vi "串口上位机.vi"() -> ()   [LabVIEW 2011]
uses:
  <vilib>/Utility/error.llb/whitespace.ctl
  <vilib>/Instr/_visa.llb/VISA Configure Serial Port (Instr).vi
  <vilib>/Utility/file.llb/Write To Spreadsheet File (string).vi
panel:
  out "提示灯":bool
  out "连接的字符串":string
  out "心率记录表":string[][](table)
  in  "心率文档存放路径":path
  out "错误输出":errorcluster
  out "接收手机端内容显示区":string
  out "错误输出 2":errorcluster caption="错误输出"
  in  "停止":bool
  out "心率显示":i32
  in  "确定按钮":dbl
  out "error out":errorcluster caption="错误输出"
  out "滑动杆":T1 scale=0.0..10.0
  out "发送记录":string
  out "发送总字节数":u32
  out "发送字节数":u32
  out "发送错误状态":bool
  in  "发送":bool
  out "接收内容":string
  in  "发送内容":string
  out "工作状态":bool
  in  "baud rate (9600)":u32=115200 caption="波特率"
  in  "串口号":refnum<visa-resource-name>
  in  "关闭串口":bool
  in  "打开串口":bool
  # "嵌入式设备通信区"
  # "物联网通信区"
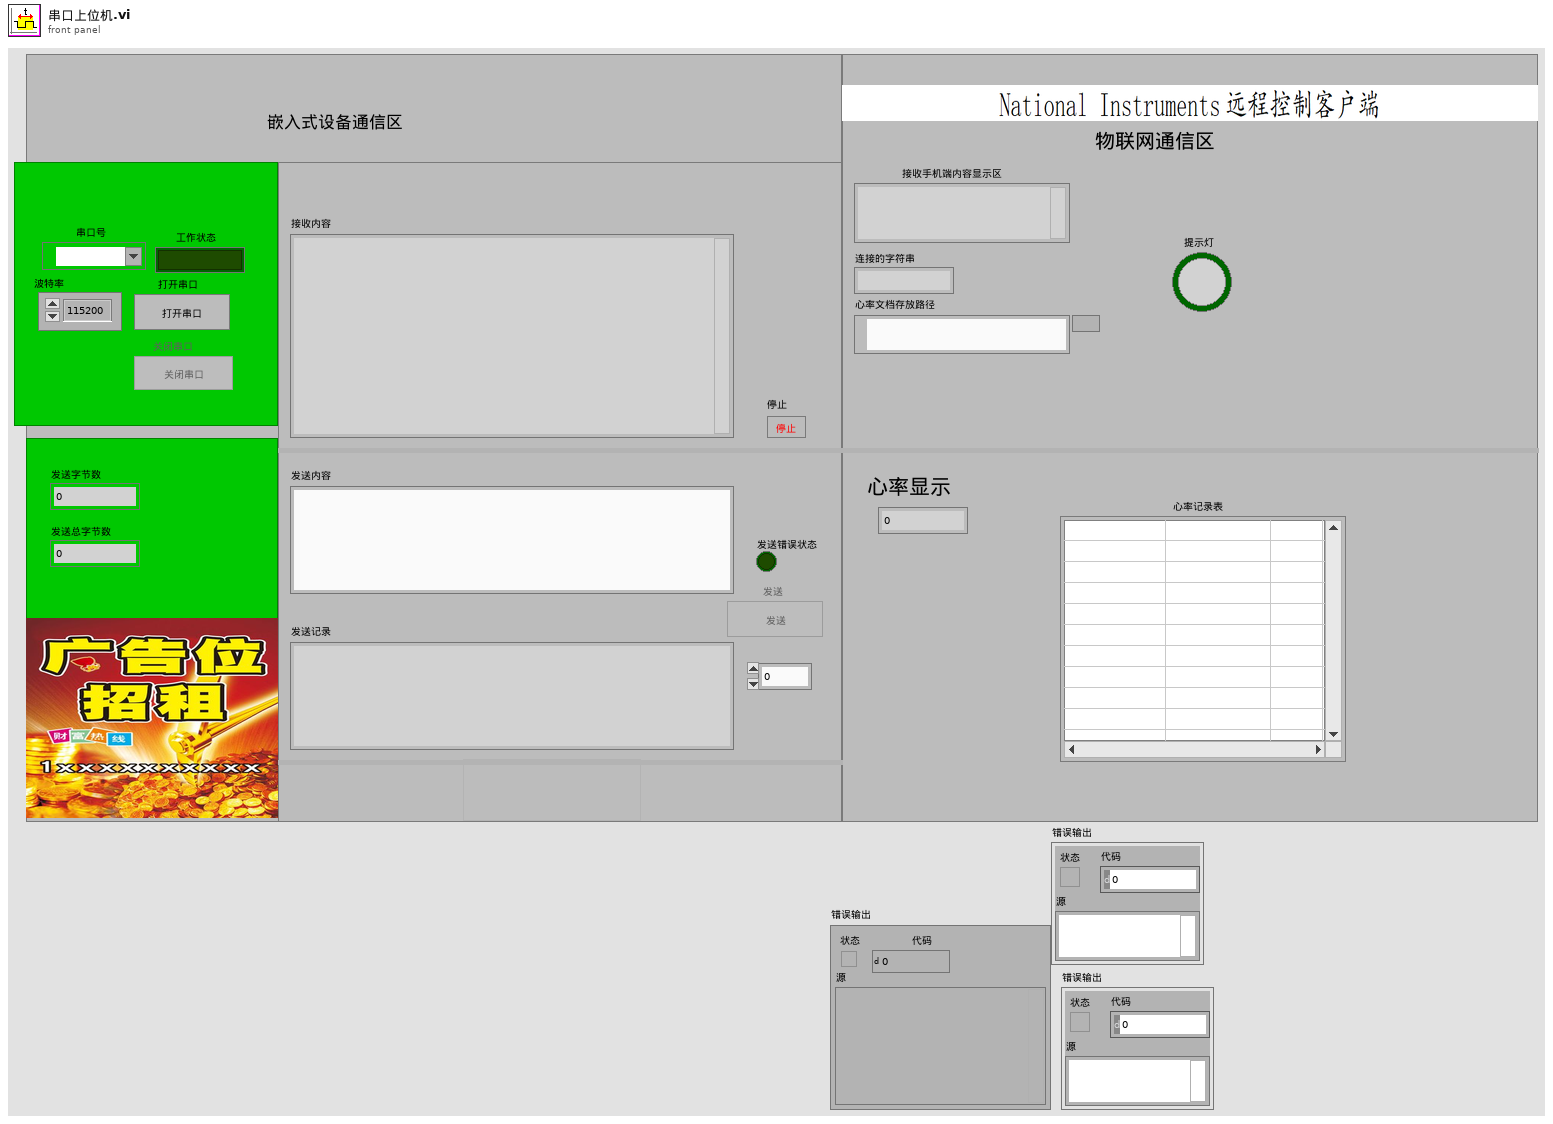
[diagram p1: front panel]
types:
  T1 = typedef "滚动条.ctl" = dbl
  T2 = enum8{"Enabled", "Disabled", "Disabled and Grayed Out"}
  T3 = typedef "whitespace.ctl" = u16
  T4 = enum16{"Standard", "Buffered", "CRLF", "Immediate"}
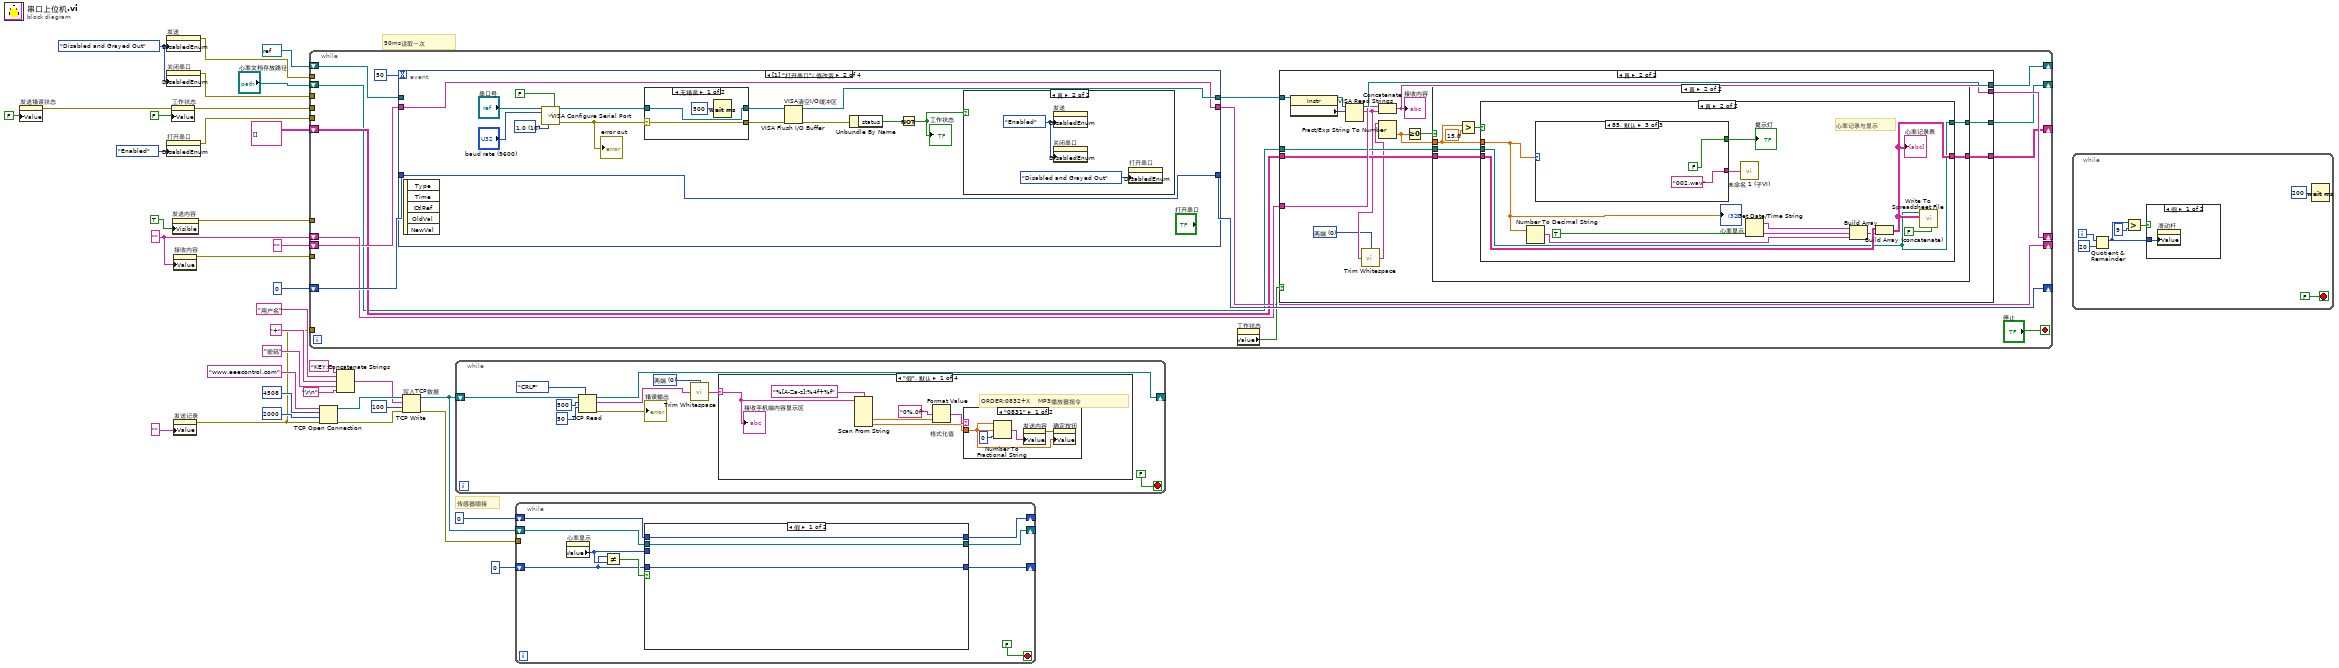
[diagram p0: block diagram]
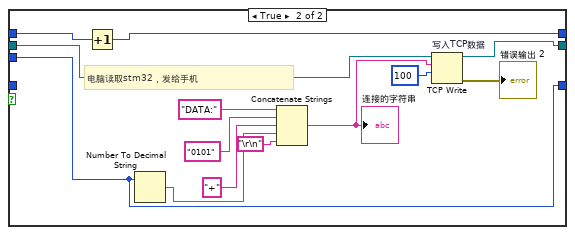
[diagram p6: hidden frame]
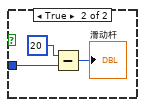
[diagram p7: hidden frame]
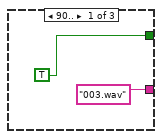
[diagram p11: hidden frame]
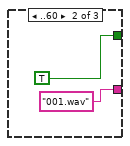
[diagram p12: hidden frame]
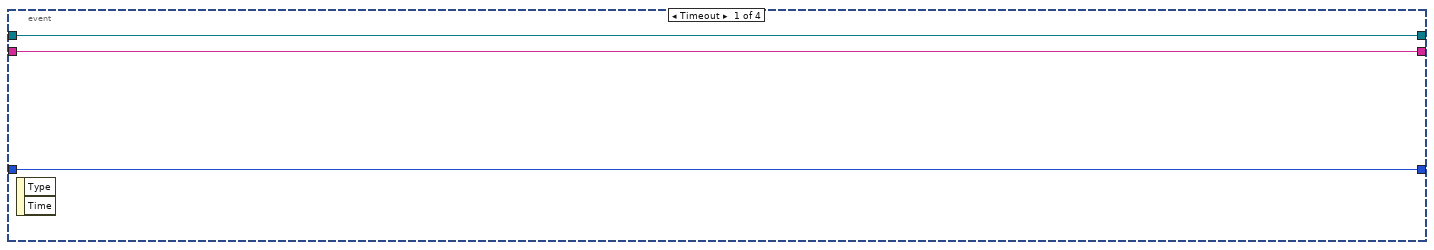
[diagram p13: hidden frame]
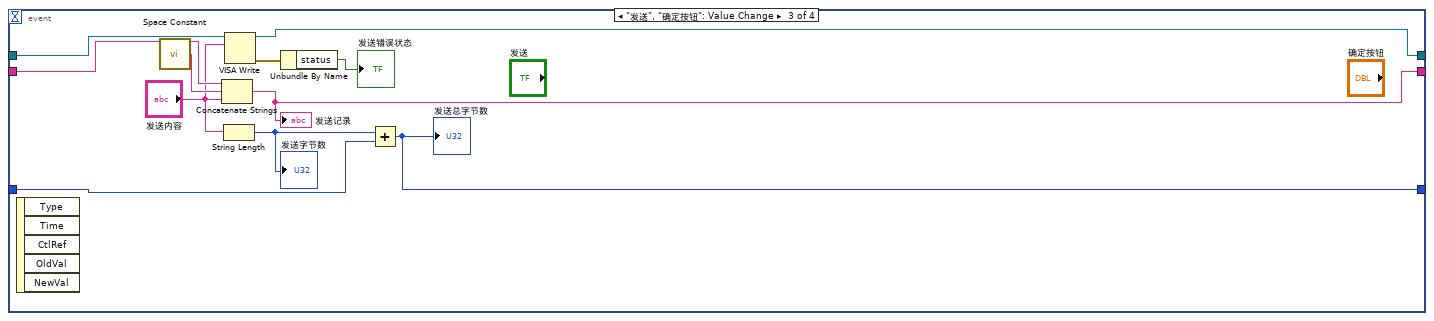
[diagram p16: hidden frame]
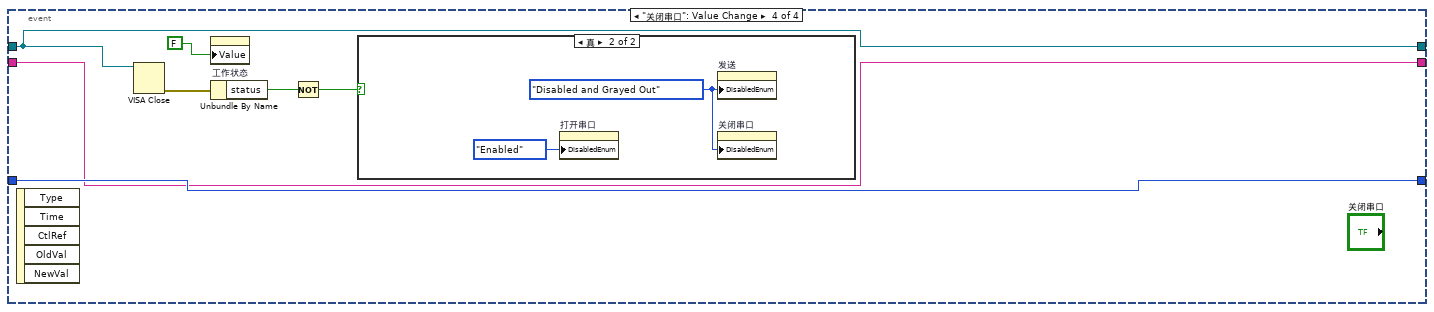
[diagram p17: hidden frame]
diagram:
  w7 = ""
  w31 = T2."Disabled and Grayed Out" ("禁用")
  # "传感器顺接"
  # "50ms读取一次"
  n1 = property on="发送错误状态" class="Bool (严格)"("Value"=FALSE ("发送错误状态")) -> (error out=w29:errorcluster)  [unwired: 2 in, 1 out]
  n2 = property on="发送" class="Bool"("DisabledEnum"=w31) -> (error out=w32:errorcluster)  [unwired: 2 in, 1 out]
  n3 = property on="关闭串口" class="Bool"("DisabledEnum"=w31) -> (error out=w34:errorcluster)  [unwired: 2 in, 1 out]
  n4 = property on="打开串口" class="Bool"("DisabledEnum"=T2."Enabled" ("禁用")) -> (error out=w35:errorcluster)  [unwired: 2 in, 1 out]
  n5 = property on="工作状态" class="Bool (严格)"(error in=w29, "Value"=FALSE ("工作状态")) -> (error out=w30:errorcluster)  [unwired: 1 in, 1 out]
  n6 = property on="发送内容" class="Str"("Visible"=TRUE ("可见")) -> (error out=w24:errorcluster)  [unwired: 2 in, 1 out]
  n7 = property on="接收内容" class="Str"("Value"=w7) -> (error out=w8:errorcluster)  [unwired: 2 in, 1 out]
  n8 = property on="发送记录" class="Str"("Value"="" ("发送记录")) -> (error out=w6:errorcluster)  [unwired: 2 in, 1 out]
  n9 = while {
    shift-right: [w46] -> _
    shift-left: refnum<visa-resource-name> refnum ("VISA resource name out") -> [w51]
    tunnel: w35 -> [_]
    tunnel: w34 -> [_]
    tunnel: w32 -> [_]
    tunnel: w30 -> [_]
    shift-right: [w50] -> _
    shift-left: 0 -> [w49]
    shift-right: [w45] -> _
    shift-left: w7 -> [w44]
    tunnel: w24 -> [_]
    shift-right: [w42] -> _
    shift-left: "" -> [w43]
    tunnel: w6 -> [_]
    tunnel: w8 -> [_]
    shift-right: [w39] -> _
    shift-left: string[][] [] -> [w40]
    shift-right: [w37] -> _
    shift-left: "心率文档存放路径" -> [w38]
    stop <- "停止" stop-if-true
    n10 = event shown="[1] \"打开串口\": 值改变" {
      selector: _ -> [_ _ _ _]
      dyn-events: _ -> [_ _ _ _]
      timeout: 50 -> [_ _ _ _]
      tunnel: [w102 w108 w134 w136] -> w47
      tunnel: w51 -> [w102 _ w135 w136]
      tunnel: [w103 w106 w130 w139] -> w50
      tunnel: w49 -> [w103 w106 w129 w139]
      tunnel: w43 -> [w101 w105 w128 w137]
      tunnel: [w101 w105 w125 w137] -> w42
      event Timeout {
        n11 = event-data() -> ()  [unwired: 1 in, 2 out]
      }
      event "打开串口": Value Change {
        w104 = u16 10 items=["1.0"=10, "1.5"=15, "2.0"=20] ("stop bits (10: 1 bit)")
        n12 = event-data() -> ()  [unwired: 1 in, 5 out]
        n13 = call-poly "VISA Configure Serial Port"("VISA resource name"="串口号", "Enable Termination\nChar (T)"=FALSE ("Enable Termination\nChar (T)"), "baud rate (9600)"="baud rate (9600)", "stop bits (10: 1 bit)"=w104) -> ("VISA resource name out"=w111:refnum<visa-resource-name>, "error out"=w114:errorcluster)  [unwired: 10 in]
        "error out" <- w114
        n14 = case shown="无错误" w114 {
          selector: w114 -> [w121 w124]
          tunnel: [w121 w124] -> w113
          tunnel: w111 -> [w120 w123]
          tunnel: [w120 w123] -> w112
          frame No Error {
            n15 = Wait (ms)(milliseconds to wait=u32 500 ("等待时间（毫秒）")) -> ()  [unwired: 1 out]
          }
          frame Error {
          }
        }
        n16 = VISA Flush I/O Buffer "VISA清空I/O缓冲区"(VISA resource name=w112, error in (no error)=w113) -> (VISA resource name out=w108:refnum<visa-resource-name>, error out=w110:errorcluster)  [unwired: 1 in]
        n17 = Unbundle By Name(w110) -> ("status"=w109:bool)
        n18 = Not(x=w109) -> (.not. x?=w107:bool)
        "工作状态" <- w107
        n19 = case shown="真" w107 {
          frame False {
          }
          frame True {
            w118 = T2."Enabled" ("禁用")
            n20 = property on="发送" class="Bool"("DisabledEnum"=w118) -> ()  [unwired: 2 in, 2 out]
            n21 = property on="关闭串口" class="Bool"("DisabledEnum"=w118) -> ()  [unwired: 2 in, 2 out]
            n22 = property on="打开串口" class="Bool"("DisabledEnum"=T2."Disabled and Grayed Out" ("禁用")) -> ()  [unwired: 2 in, 2 out]
          }
        }
      }
      event "发送", "确定按钮": Value Change {
        n23 = event-data() -> ()  [unwired: 1 in, 5 out]
        n24 = call <vilib>:"Space Constant.vi"() -> ("String"=w127:string)
        n25 = Concatenate Strings(w128, w127, "发送内容") -> (w125:string)
        "发送记录" <- w125
        n26 = String Length(string="发送内容") -> (length=w131:i32)
        "发送字节数" <- w131
        n27 = VISA Write(VISA resource name=w135, write buffer="发送内容") -> (VISA resource name out=w134:refnum<visa-resource-name>, error out=w133:errorcluster)  [unwired: 1 in, 1 out]
        n28 = Unbundle By Name(w133) -> ("status"=→"发送错误状态":bool)
        n29 = Add(x=w131, y=w129) -> (x+y=w130:i32)
        "发送总字节数" <- w130
      }
      event "关闭串口": Value Change {
        n30 = event-data() -> ()  [unwired: 1 in, 5 out]
        n31 = VISA Close(VISA resource name=w136) -> (error out=w142:errorcluster)  [unwired: 1 in]
        n32 = property on="工作状态" class="Bool (严格)"("Value"=FALSE ("工作状态")) -> ()  [unwired: 2 in, 2 out]
        n33 = Unbundle By Name(w142) -> ("status"=w141:bool)
        n34 = Not(x=w141) -> (.not. x?=w140:bool)
        n35 = case shown="真" w140 {
          frame False {
          }
          frame True {
            w143 = T2."Disabled and Grayed Out" ("禁用")
            n36 = property on="打开串口" class="Bool"("DisabledEnum"=T2."Enabled" ("禁用")) -> ()  [unwired: 2 in, 2 out]
            n37 = property on="发送" class="Bool"("DisabledEnum"=w143) -> ()  [unwired: 2 in, 2 out]
            n38 = property on="关闭串口" class="Bool"("DisabledEnum"=w143) -> ()  [unwired: 2 in, 2 out]
          }
        }
      }
    }
    n39 = property on="工作状态" class="Bool (严格)"() -> ("Value"=w48:bool)  [unwired: 2 in, 2 out]
    n40 = case shown="真" w48 {
      tunnel: w47 -> [w56 w69]
      tunnel: [w56 w68] -> w46
      tunnel: [w55 w66] -> w45
      tunnel: w44 -> [w55 w67]
      tunnel: w40 -> [w54 w65]
      tunnel: [w54 w64] -> w39
      tunnel: w38 -> [w53 w63]
      tunnel: [w53 w62] -> w37
      frame False {
      }
      frame True {
        w57 = T3 0 items=["两端", "字符串首端", "字符串末端"] ("location (both)")
        n41 = property class="Instr"(reference=w69) -> (reference out=w71:refnum<visa-resource-name>, "Serial Settings:Number of Bytes at Serial Port"=w70:u32)  [unwired: 1 in, 1 out]
        n42 = VISA Read(VISA resource name=w71, byte count=w70) -> (VISA resource name out=w68:refnum<visa-resource-name>, read buffer=w59:string)  [unwired: 1 in, 2 out]
        n43 = call <vilib>:"Trim Whitespace.vi"("string"=w59, "location (both)"=w57) -> ("trimmed string"=w58:string)
        n44 = Concatenate Strings(w67, w59) -> (w66:string)
        "接收内容" <- w66
        n45 = Fract/Exp String To Number ("分数/指数字符串至数值转换")(string=w58) -> (number=w60:dbl)  [unwired: 3 in, 1 out]
        n46 = Greater Or Equal To 0?(x=w60) -> (x >= 0?=w61:bool)
        n47 = case shown="真" w61 {
          tunnel: w60 -> [_ w74]
          tunnel: w65 -> [w73 w80]
          tunnel: [w73 w79] -> w64
          tunnel: w63 -> [w72 w78]
          tunnel: [w72 w75] -> w62
          frame False {
          }
          frame True {
            n48 = Greater?(x=w74, y=15.0) -> (0:w76:bool)
            n49 = case shown="真" w76 {
              tunnel: w80 -> [w82 w92]
              tunnel: [w82 w87] -> w79
              tunnel: w78 -> [w81 w86]
              tunnel: w74 -> [_ w84]
              tunnel: [w81 w86] -> w75
              frame False {
              }
              frame True {
                # "心率记录与显示"
                n50 = Number To Decimal String ("数值至十进制数字符串转换")(number=w84) -> (decimal integer string=w89:string)  [unwired: 1 in]
                n51 = case shown="85, 默认" w84 {
                  tunnel: [TRUE TRUE FALSE] -> w85
                  tunnel: ["003.wav" "001.wav" "002.wav"] -> w83
                  frame 90.. {
                  }
                  frame ..60 {
                  }
                  frame 85, Default {
                  }
                }
                "提示灯" <- w85
                n52 = call "未命名 1 (子VI).vi"("字符串"=w83) -> ()  [unwired: 1 in]
                n53 = Get Date/Time String(want seconds? (F)=TRUE ("需要秒？(F)")) -> (date string=w91:string, time string=w90:string)  [unwired: 2 in]
                n54 = Build Array(w91, w90, w89) -> (w88:string[])
                n55 = Build Array (concatenate)(w92, w88) -> (w87:string[][])
                "心率记录表" <- w87
                n56 = call-poly <vilib>:"Write To Spreadsheet File.vi"("transpose? (no:F)"=FALSE, "2D data"=w87, "file path (dialog if empty)"=w86) -> ()  [unwired: 5 in, 1 out]
                "心率显示" <- w84
              }
            }
          }
        }
      }
    }
  }
  n57 = TCP Open Connection(address="www.eeecontrol.com" ("地址"), remote port or service name=u16 4508 ("远程端口或服务名称"), timeout ms (60000)=2000 ("超时毫秒(60000)"), error in (no error)=w6) -> (connection ID=w18:refnum<k5>, error out=w16:errorcluster)  [unwired: 1 in]
  n58 = Concatenate Strings("KEY:" ("字符串"), "用户名" ("字符串"), "+" ("字符串"), "密码" ("字符串"), "\r\n") -> (w10:string)
  n59 = TCP Write "写入TCP数据"(connection ID=w18, data in=w10, error in (no error)=w16, 9:100 ("超时毫秒(25000)")) -> (connection ID out=w4:refnum<k5>, error out=w17:errorcluster)  [unwired: 1 out]
  n60 = while {
    shift-right: [w147] -> _
    shift-left: w4 -> [w154]
    stop <- FALSE stop-if-true
    w149 = T3 0 items=["两端", "字符串首端", "字符串末端"] ("location (both)")
    n61 = TCP Read(connection ID=w154, bytes to read=500 ("读取的字节"), 7:T4."CRLF" ("模式（标准）"), 9:50 ("超时毫秒(25000)")) -> (connection ID out=w147:refnum<k5>, data out=w150:string, error out=→"错误输出":errorcluster)  [unwired: 1 in]
    n62 = call <vilib>:"Trim Whitespace.vi"("string"=w150, "location (both)"=w149) -> ("trimmed string"=w148:string)
    n63 = case shown="\"假\", 默认" w148 {
      selector: w148 -> [w160 _ _ _]
      frame "假", Default {
        # "ORDER:0832+X    MP3播放器指令"
        n64 = Scan From String(format string="%[A-Za-z]:%4f+%f" ("格式字符串"), input string=w160) -> (output 2=w157:dbl, output 3=w155:dbl)  [unwired: 6 in, 3 out]
        n65 = Format Value "格式化值"(format string="0%.0f" ("格式字符串"), value (0)=w157) -> (output string=w156:string)  [unwired: 1 in]
        n66 = case shown="\"0831\"" w156 {
          tunnel: w155 -> [w161 _]
          frame "0831" {
            n67 = Number To Fractional String(number=w161, width (-)=w161, precision (6)=i16 0 ("精度(6)")) -> (F-format string=w163:string)  [unwired: 1 in]
            n68 = property on="发送内容" class="Str"("Value"=w163) -> (error out=w162:errorcluster)  [unwired: 2 in, 1 out]
            n69 = property on="确定按钮" class="DigNum (严格)"(error in=w162, "Value"=w161) -> ()  [unwired: 1 in, 2 out]
          }
          frame "0", Default {
          }
        }
        "接收手机端内容显示区" <- w160
      }
      frame "" {
      }
      frame "PING" {
      }
      frame "STATE:login-success" {
      }
    }
  }
  n70 = while {
    shift-right: [w171] -> _
    shift-left: w4 -> [w172]
    tunnel: w17 -> [_]
    shift-right: [w170] -> _
    shift-left: 0 -> [w165]
    shift-right: [w166] -> _
    shift-left: 0 -> [w167]
    stop <- FALSE stop-if-true
    n71 = property on="心率显示" class="DigNum (严格)"() -> ("Value"=w169:i32)  [unwired: 2 in, 2 out]
    n72 = Not Equal?(x=w165, y=w169) -> (x != y?=w168:bool)
    n73 = case shown="假" w168 {
      tunnel: w172 -> [w176 w189]
      tunnel: [w176 w188] -> w171
      tunnel: w169 -> [_ w180]
      tunnel: [w174 w180] -> w170
      tunnel: w167 -> [w175 w179]
      tunnel: [w175 w178] -> w166
      tunnel: w165 -> [w174 _]
      frame False {
      }
      frame True {
        # "电脑读取stm32，发给手机"
        n74 = Increment(x=w179) -> (x+1=w178:i32)
        n75 = Number To Decimal String(number=w180) -> (decimal integer string=w183:string)  [unwired: 1 in]
        n76 = Concatenate Strings("DATA:" ("字符串"), "0101", "+" ("字符串"), w183, "\r\n") -> (w186:string)
        "连接的字符串" <- w186
        n77 = TCP Write "写入TCP数据"(connection ID=w189, data in=w186, 9:100 ("超时毫秒(25000)")) -> (connection ID out=w188:refnum<k5>, error out=→"错误输出 2":errorcluster)  [unwired: 1 in, 1 out]
      }
    }
  }
  n78 = while {
    i -> [w193]
    stop <- FALSE stop-if-true
    n79 = Quotient & Remainder(x=w193, y=20) -> (x-y*floor(x/y)=w190:i32)  [unwired: 1 out]
    n80 = Greater?(x=w190, y=9) -> (0:w191:bool)
    n81 = case shown="假" w191 {
      tunnel: w190 -> [w197 w199]
      frame False {
        n82 = property on="滑动杆" class="Slide (严格)"("Value"=w197) -> ()  [unwired: 2 in, 2 out]
      }
      frame True {
        n83 = Subtract(x=20 ("y"), y=w199) -> (x-y=→"滑动杆":i32)
      }
    }
    n84 = Wait (ms)(milliseconds to wait=u32 200 ("等待时间（毫秒）")) -> ()  [unwired: 1 out]
  }
